vi "criteria_count.vi"(8 "error in (no error)":errorcluster, 10 "recipe_data":variant, 11 "criteria":variant) -> (0 "error out":errorcluster)   [LabVIEW 2015, in "example_01.lvlib"]
uses:
  example_01.lvlib
  _controls/recipes.ctl
  _controls/steps_actions_data.ctl
  _controls/steps_actions.ctl
  <userlib>/antonio-alexander/lv-recipe-machine/lv-recipe-machine.lvlib
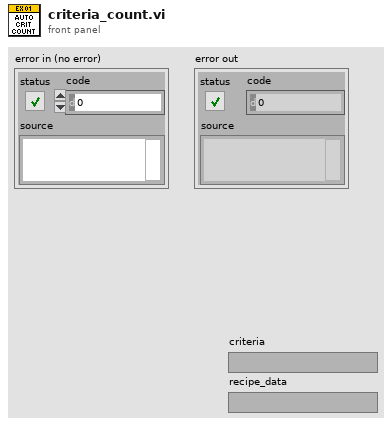
[diagram p1: front panel]
types:
  T1 = typedef "example_01.lvlib/recipes.ctl" = enum16{"<recipes>", "wait_random", "random_wait", "count", "comparison", "launch", "<null>"}
  T2 = typedef "example_01.lvlib/steps_actions.ctl" = enum16{"<steps_actions>", "manual_random", "manual_comparison", "manual_wait", "auto_random", "auto_wait", "criteria_initialize", "criteria_count", "criteria_comparison", "transition_simple", "transition_count", "transition_comparison", "launch_wait", "<null>"}
  T3 = typedef "example_01.lvlib/steps_actions_data.ctl" = cluster{"step_action":T2, "data":variant}
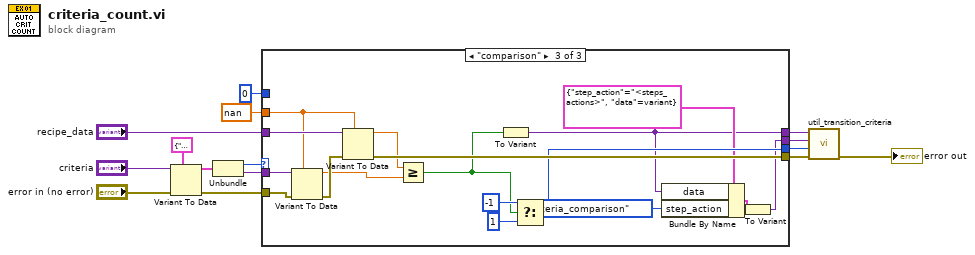
[diagram p0: block diagram]
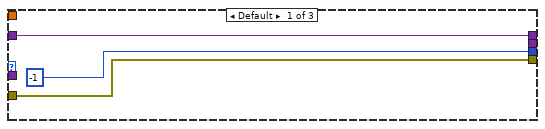
[diagram p2: hidden frame]
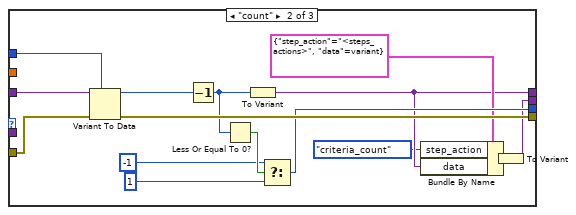
[diagram p3: hidden frame]
diagram:
  n1 = Variant To Data(error in="error in (no error)", type=cluster{"recipe":T1, variant} {"recipe"=enum."<recipes>", variant}, Variant="criteria") -> (data=w13:cluster{"recipe":T1, variant}, error out=w9:errorcluster)
  n2 = Unbundle(w13) -> ("recipe"=w11:T1, w3:variant)
  n3 = case shown="\"comparison\"" w11 {
    tunnel: w9 -> [w17 w29 w44]
    tunnel: "recipe_data" -> [w18 w33 w50]
    tunnel: [w18 w22 w35] -> w4
    tunnel: [w17 w32 w49] -> w5
    tunnel: 0 -> [_ w31 _]
    tunnel: nan -> [_ _ w43]
    tunnel: w3 -> [_ _ w45]
    tunnel: [-1 w27 w48] -> w2
    tunnel: [_ w19 w36] -> w1
    frame Default {
    }
    frame "count" {
      n4 = Variant To Data(error in=w29, type=w31, Variant=w33) -> (data=w30:i32, error out=w32:errorcluster)
      n5 = Decrement(x=w30) -> (x-1=w28:i32)
      n6 = Less Or Equal To 0?(x=w28) -> (x <= 0?=w26:bool)
      n7 = To Variant(anything=w28) -> (Variant=w22:variant)
      n8 = Select(t=-1, s=w26, f=1) -> (s? t:f=w27:i32)
      n9 = Bundle By Name(cluster=T3 {"step_action"=enum."<steps_actions>", "data"=variant} ("step_data"), "step_action"=steps_actions."criteria_count", "data"=w22) -> (w20:T3)
      n10 = To Variant(anything=w20) -> (Variant=w19:variant)
    }
    frame "comparison" {
      n11 = Variant To Data(error in=w44, type=w43, Variant=w45) -> (data=w40:dbl, error out=w42:errorcluster)
      n12 = Variant To Data(error in=w42, type=w43, Variant=w50) -> (data=w41:dbl, error out=w49:errorcluster)
      n13 = Greater Or Equal?(x=w41, y=w40) -> (x >= y?=w39:bool)
      n14 = To Variant(anything=w39) -> (Variant=w35:variant)
      n15 = Select(t=-1, s=w39, f=1) -> (s? t:f=w48:i32)
      n16 = Bundle By Name(cluster=T3 {"step_action"=enum."<steps_actions>", "data"=variant} ("step_data"), "data"=w35, "step_action"=steps_actions."criteria_comparison") -> (w37:T3)
      n17 = To Variant(anything=w37) -> (Variant=w36:variant)
    }
  }
  n18 = call <userlib>:"util_transition_criteria.vi"("error in (no error)"=w5, "next_index"=w2, "data"=w1, "recipe_data"=w4) -> ("error out"=→"error out":errorcluster)  [unwired: 7 in]
